vi "Fake VTI module.vi"(8 "Top address in":T1, 11 "VTI Module ref":T2) -> ()   [LabVIEW 2021, in "Temperature controller.lvlib"]
uses:
  Temperature controller.lvlib
  Messenger service/Data types/Modul ref.ctl
  Messenger service/Data types/Mailbox address.ctl
  Messenger service/Data types/Module name.ctl
  ctl/TC sensors.ctl
  ctl/Set temperature.ctl
  ctl/MSG for VTI.ctl
  ctl/TC commands.ctl
  Messenger service/MessengerLib.lvlib
panel:
  out "1 run\n time":u32
  out "TC port":refnum<visa-resource-name>
  out "Initialized?":bool
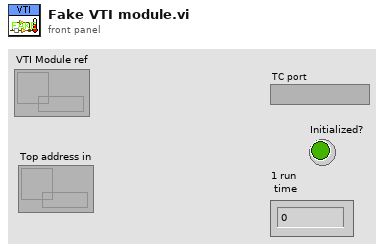
[diagram p1: front panel]
types:
  T1 = typedef "MessengerLib.lvlib/Mailbox address.ctl" = refnum<queue>
  T2 = typedef "MessengerLib.lvlib/Modul ref.ctl" = refnum<queue>
  T3 = typedef "Module name.ctl" = enum16{"Emty", "Magnet", "VTI", "Excitation", "Servo", "Acquisition", "Rotator", "Digitizer", "SMU2450", "Carousel", "Multimeter", "Tmp monitor", "Power monitor"}
  T4 = typedef "Temperature controller.lvlib/TC sensors.ctl" = cluster{"VTI space":dbl, "Sample":dbl, "He pot":dbl, "Trap":dbl, "Ambient":dbl, "SetP_VTI":dbl, "SetP_Smp":dbl, "SetP_Pot":dbl, "SetP_Trap":dbl, "Range out 1":u16, "Out 1 [%]":dbl, "Out 2 [%]":dbl}
  T5 = typedef "Temperature controller.lvlib/Set temperature.ctl" = cluster{"VTI space [K]":dbl, "Sample [K]":dbl, "Heater3 [K]":dbl, "Heater4 [K]":dbl, "Out 1 [%]":dbl, "Out 2 [%]":dbl, "Range out 1":u16}
  T6 = typedef "Temperature controller.lvlib/TC commands.ctl" = enum16{"Initialize", "Update", "Stop tmp change", "Set temperature", "Set point", "Disconnect", "End", "Ignore"}
  T7 = typedef "Temperature controller.lvlib/MSG for VTI.ctl" = cluster{"Command":T6, "Data":variant}
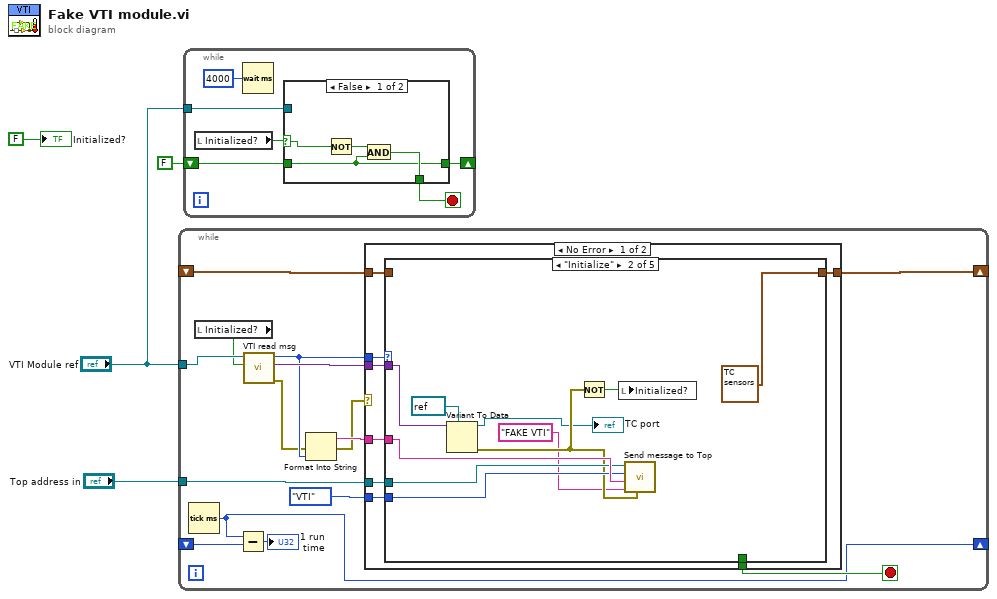
[diagram p0: block diagram]
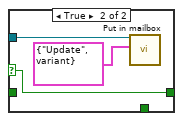
[diagram p2: hidden frame]
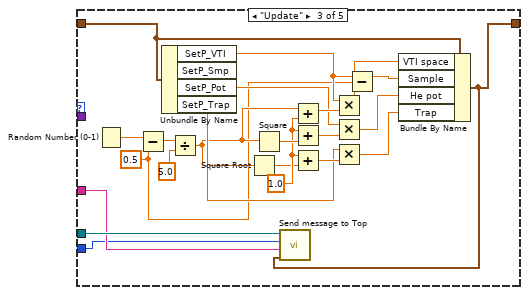
[diagram p4: hidden frame]
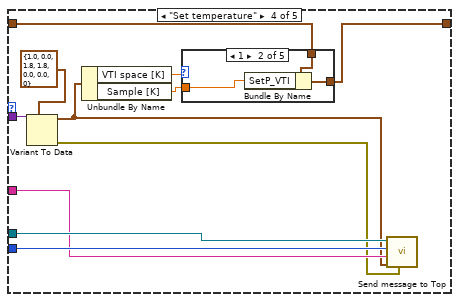
[diagram p5: hidden frame]
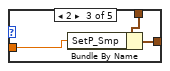
[diagram p7: hidden frame]
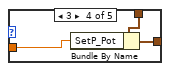
[diagram p8: hidden frame]
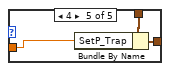
[diagram p9: hidden frame]
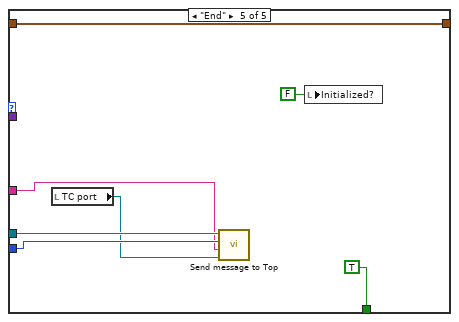
[diagram p10: hidden frame]
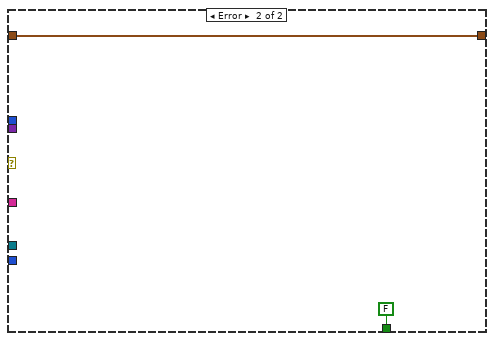
[diagram p11: hidden frame]
diagram:
  n1 = while {
    tunnel: "VTI Module ref" -> [w17]
    tunnel: "Top address in" -> [w18]
    shift-right: [w9] -> _
    shift-left: _ -> [w13]
    shift-right: [w12] -> _
    shift-left: _ -> [w11]
    stop <- w14 stop-if-true
    n2 = Tick Count (ms)() -> (millisecond timer value=w12:u32)
    n3 = local read "Initialized?"() -> (w8:bool)
    n4 = Subtract(x=w12, y=w11) -> (x-y=→"1 run\n time":u32)
    n5 = call "VTI read msg.vi"("Initialized?"=w8, "Queue in"=w17) -> ("error out"=w6:errorcluster, "Data"=w16:variant, "Command"=w7:T6)  [unwired: 6 in, 1 out]
    n6 = Format Into String(error in=w6, w7) -> (resulting string=w15:string, error out=w5:errorcluster)  [unwired: 2 in]
    n7 = case shown="No Error" w5 {
      tunnel: Module_name."VTI" ("Module name") -> [w27 _]
      tunnel: w18 -> [w26 _]
      tunnel: w16 -> [w25 _]
      tunnel: w15 -> [w24 _]
      tunnel: [w23 FALSE] -> w14
      tunnel: w13 -> [w22 w94]
      tunnel: [w21 w94] -> w9
      tunnel: w7 -> [w20 _]
      frame No Error {
        n8 = case shown="\"Initialize\"" w20 {
          tunnel: w27 -> [_ w34 w40 w72 w92]
          tunnel: w26 -> [_ w35 w61 w71 w91]
          tunnel: w25 -> [_ w37 _ w69 _]
          tunnel: w24 -> [_ w36 w60 w70 w90]
          tunnel: [_ _ _ _ TRUE] -> w23
          tunnel: [w28 T4 {"VTI space"=1.82, "Sample"=0.0, "He pot"=0.0, "Trap"=0.0, "Ambient"=0.0, "SetP_VTI"=1.8, "SetP_Smp"=4.0, "SetP_Pot"=3.8, "SetP_Trap"=8.0, "Range out 1"=1, "Out 1 [%]"=0.0, "Out 2 [%]"=0.0} ("TC sensors [K]") w39 w65 w86] -> w21
          tunnel: w22 -> [w28 _ w48 w66 w86]
          frame "Ignore", Default {
          }
          frame "Initialize" {
            n9 = Variant To Data(type=refnum<visa-resource-name> refnum ("VISA resource name"), Variant=w37) -> (data=→"TC port":refnum<visa-resource-name>, error out=w32:errorcluster)  [unwired: 1 in]
            n10 = Not(x=w32) -> (.not. x?=w33:bool)
            n11 = local write "Initialized?"(w33) -> ()
            n12 = call "Send message to Top.vi"("Error in (no error)"=w32, "Data"="FAKE VTI", "Response"=w36, "Module"=w34, "Mailbox address in"=w35) -> ()  [unwired: 5 in, 2 out]
          }
          frame "Update" {
            w41 = 0.5 ("y")
            w58 = 1.0
            n13 = Random Number (0-1)() -> (number: 0 to 1=w57:dbl)
            n14 = Subtract(x=w57, y=w41) -> (x-y=w47:dbl)
            n15 = Unbundle By Name(w48) -> ("SetP_VTI"=w43:dbl, "SetP_Pot"=w53:dbl, "SetP_Trap"=w52:dbl)  [unwired: 1 out]
            n16 = Divide(x=w47, y=5.0) -> (x/y=w46:dbl)
            n17 = Square Root(x=w46) -> (sqrt(x)=w44:dbl)
            n18 = Square(x=w46) -> (x^2=w59:dbl)
            n19 = Add(x=w46, y=w58) -> (x+y=w54:dbl)
            n20 = Add(x=w58, y=w59) -> (x+y=w56:dbl)
            n21 = Add(x=w58, y=w44) -> (x+y=w55:dbl)
            n22 = Multiply(x=w43, y=w54) -> (x*y=w49:dbl)
            n23 = Multiply(x=w53, y=w56) -> (x*y=w50:dbl)
            n24 = Multiply(x=w52, y=w55) -> (x*y=w51:dbl)
            n25 = Subtract(x=w43, y=w41) -> (x-y=w42:dbl)
            n26 = Bundle By Name(cluster=w48, "VTI space"=w49, "Sample"=w42, "He pot"=w50, "Trap"=w51) -> (w39:T4)
            n27 = call "Send message to Top.vi"("Data"=w39, "Response"=w60, "Module"=w40, "Mailbox address in"=w61) -> ()  [unwired: 6 in, 2 out]
          }
          frame "Set temperature" {
            n28 = Variant To Data(type=T5 {"VTI space [K]"=1.0, "Sample [K]"=0.0, "Heater3 [K]"=1.8, "Heater4 [K]"=1.8, "Out 1 [%]"=0.0, "Out 2 [%]"=0.0, "Range out 1"=0}, Variant=w69) -> (data=w64:T5, error out=w67:errorcluster)  [unwired: 1 in]
            n29 = Unbundle By Name(w64) -> ("VTI space [K]"=w63:dbl, "Sample [K]"=w62:dbl)
            n30 = case shown="1" w63 {
              tunnel: w66 -> [w73 w76 w79 w82 w85]
              tunnel: [w73 w75 w78 w81 w84] -> w65
              tunnel: w62 -> [_ w74 w77 w80 w83]
              frame 0, Default {
              }
              frame 1 {
                n31 = Bundle By Name(cluster=w76, "SetP_VTI"=w74) -> (w75:T4)
              }
              frame 2 {
                n32 = Bundle By Name(cluster=w79, "SetP_Smp"=w77) -> (w78:T4)
              }
              frame 3 {
                n33 = Bundle By Name(cluster=w82, "SetP_Pot"=w80) -> (w81:T4)
              }
              frame 4 {
                n34 = Bundle By Name(cluster=w85, "SetP_Trap"=w83) -> (w84:T4)
              }
            }
            n35 = call "Send message to Top.vi"("Error in (no error)"=w67, "Data"=w64, "Response"=w70, "Module"=w72, "Mailbox address in"=w71) -> ()  [unwired: 5 in, 2 out]
          }
          frame "End" {
            n36 = local read "TC port"() -> (w87:refnum<visa-resource-name>)
            n37 = call "Send message to Top.vi"("Data"=w87, "Response"=w90, "Module"=w92, "Mailbox address in"=w91) -> ()  [unwired: 6 in, 2 out]
            n38 = local write "Initialized?"(FALSE ("Initialized?")) -> ()
          }
        }
      }
      frame Error {
      }
    }
  }
  n39 = while {
    tunnel: "VTI Module ref" -> [w98]
    shift-right: [w97] -> _
    shift-left: FALSE -> [w96]
    stop <- w95 stop-if-true
    n40 = local read "Initialized?"() -> (w99:bool)
    n41 = Wait (ms)(milliseconds to wait=u32 4000) -> ()  [unwired: 1 out]
    n42 = case shown="False" w99 {
      selector: w99 -> [w104 w105]
      tunnel: w98 -> [_ w107]
      tunnel: [w101 w105] -> w97
      tunnel: w96 -> [w101 _]
      tunnel: [w102 _] -> w95
      frame False {
        n43 = Not(x=w104) -> (.not. x?=w103:bool)
        n44 = And(x=w103, y=w101) -> (x .and. y?=w102:bool)
      }
      frame True {
        n45 = call "Put in mailbox.vi"("Message"=T7 {"Command"=enum."Update", "Data"=variant}, "Queue in"=w107) -> ()  [unwired: 7 in, 3 out]
      }
    }
  }
  "Initialized?" <- FALSE ("Initialized?")
